vi "mod_Create Continuous QAM.vi"(0 "Symbol Rate, Hz":dbl format="%.2f", 1 "QAM system parameters":T3 {"symbol map" format="%.3f"}, 2 "PN Sequence Order":i32, 5 "bits/symbol":i32, 7 "TX Filter":T1(ring), 9 "Alpha":dbl format="%.2f", 11 "error in (no error)":errorcluster, 13 "Filter Length":i32) -> (4 "output complex waveform":T2 {"Y" format="%.3f"; "dt" format="%^.2e"; "t0" format="%.4f"}, 15 "error out":errorcluster)   [LabVIEW 2020, in "niDMT.lvlib"]
uses:
  <vilib>/addons/Modulation/niDMT.lvlib
  <vilib>/addons/Modulation/Digital/Support/Controls/QAM System Parameters.ctl
  <vilib>/addons/Modulation/Analog/controls/Complex Data Waveform.ctl
  <vilib>/addons/Modulation/Analog/support/mod_Set Error Source.vi
  <vilib>/addons/Modulation/Digital/Support/Common/Validators/mod_Generate Bits Validate.vi
  <vilib>/addons/Modulation/Digital/General/subVIs/mod_Generate Bits Pattern.vi
  <vilib>/addons/Modulation/Digital/Support/Common/Validators/mod_Generate Filter Coefficients Validate.vi
  <vilib>/addons/Modulation/Digital/General/subVIs/mod_Generate Filter Coefficients.vi
  <vilib>/addons/Modulation/Digital/General/subVIs/mod_Generate Bits PN Sequence.vi
  <vilib>/addons/Modulation/niAMT.lvlib
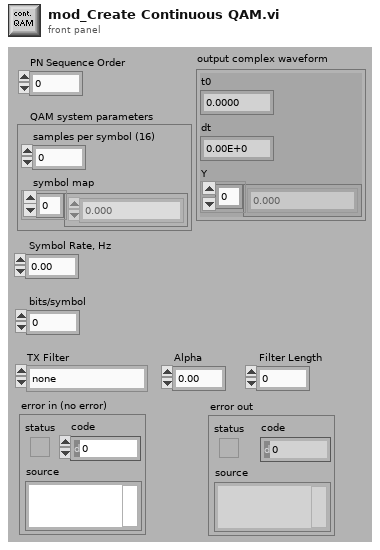
[diagram p1: front panel]
types:
  T1 = enum16{"none", "Raised Cosine", "Root Raised Cos", "Gaussian"}
  T2 = typedef "niAMT.lvlib/Complex Data Waveform.ctl" = cluster{"t0":dbl, "dt":dbl, "Y":cdb[]}
  T3 = typedef "niDMT.lvlib/QAM System Parameters.ctl" = cluster{"samples per symbol (16)":i32, "symbol map":cdb[]}
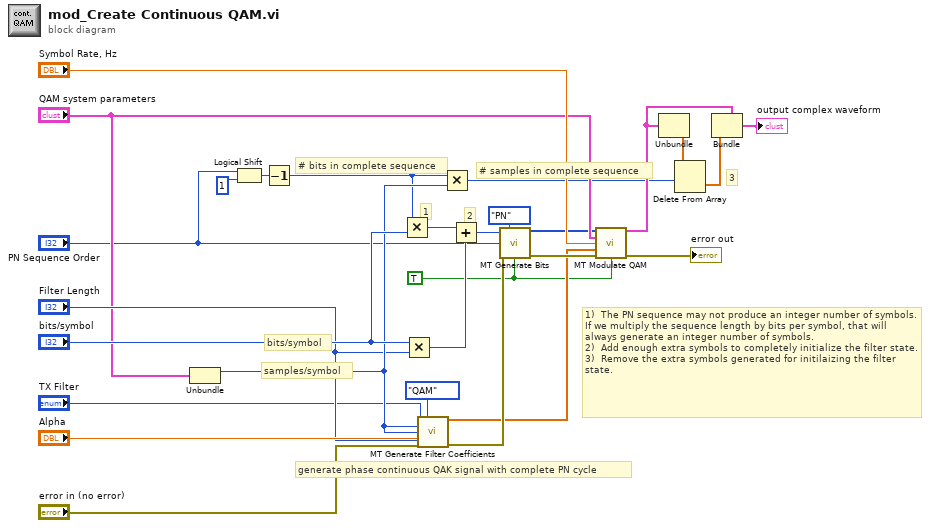
[diagram p0: block diagram]
diagram:
  w1 = TRUE ("Reset (T)")
  # "3"
  # "# samples in complete sequence"
  # "2"
  # "1"
  # "1)  The PN sequence may not produce an integer number of symbols.  If we multiply the sequence length by bits per symbol, that will always generate an integer number of symbols. \n2)  Add enough extra symbols to completely initialize the filter state.\n3)  Remove the extra symbols generated for initilaizing the filter state."
  # "# bits in complete sequence"
  # "samples/symbol"
  # "bits/symbol"
  # "generate phase continuous QAK signal with complete PN cycle"
  n1 = Unbundle("QAM system parameters") -> ("samples per symbol (16)"=w22:i32)  [unwired: 1 out]
  n2 = Logical Shift(y="PN Sequence Order", x=1) -> (x << y=w5:i32)
  n3 = Decrement(x=w5) -> (x-1=w12:i32)
  n4 = Multiply(x=w12, y="bits/symbol") -> (x*y=w7:i32)
  n5 = Multiply(x="bits/symbol", y="Filter Length") -> (x*y=w11:i32)
  n6 = call <vilib>:"MT Generate Filter Coefficients.vi"("pulse shaping filter (none)"="TX Filter", "modulation type"=enum16{"FSK", "PSK", "QAM", "MSK"}."QAM" ("Modulation Type"), "pulse shaping samples per symbol (16)"=w22, "matched samples per symbol (16)"=w22, "filter parameter"="Alpha", "error in (no error)"="error in (no error)", "filter length (symbols)"="Filter Length") -> ("pulse shaping filter coefficients"=w16:dbl[], "error out"=w25:errorcluster)  [unwired: 7 out]
  n7 = Multiply(x=w12, y=w22) -> (x*y=w14:i32)
  n8 = Add(x=w7, y=w11) -> (x+y=w8:i32)
  n9 = call <vilib>:"MT Generate Bits.vi"("total bits (128)"=w8, "mode (PN)"=enum16{"PN", "pattern", "user"}."PN" ("Mode (PN)"), "PN sequence order (9)"="PN Sequence Order", "error in (no error)"=w25, "reset? (T)"=w1) -> ("output bit stream"=w15:i8[], "error out"=w26:errorcluster)  [unwired: 3 in, 6 out]
  n10 = call <vilib>:"MT Modulate QAM.vi"("input bit stream"=w15, "QAM system parameters"="QAM system parameters", "symbol rate (Hz)"="Symbol Rate, Hz", "pulse shaping filter coefficients"=w16, "error in (no error)"=w26, "reset? (T)"=w1) -> ("output complex waveform"=w17:T2, "error out"=→"error out":errorcluster)  [unwired: 1 in, 7 out]
  n11 = Unbundle(w17) -> ("Y"=w9:cdb[])  [unwired: 2 out]
  n12 = Delete From Array(array=w9, length=w14) -> (deleted portion=w10:cdb[])  [unwired: 1 in, 1 out]
  n13 = Bundle(cluster=w17, "Y"=w10) -> (→"output complex waveform":T2)  [unwired: 2 out]
